vi "cg_Brent Search Powell.vi"(1 "p":dbl[](array[numeric]) format="%.2f", 2 "xit":dbl[](array[numeric]) format="%.2f", 3 "ZEPS":dbl=1e-12 format="%.2e", 6 "tol":dbl=1e-06 format="%.2e", 7 "function and data":T1, 8 "error in (no error)":errorcluster, 9 "c (start)":dbl=1.0 format="%.2f", 10 "b (start)":dbl=0.5 format="%.2f", 11 "a (start)":dbl format="%.2f") -> (0 "error out":errorcluster, 4 "u":dbl=1.5920119327128747e-12 format="%.2f", 5 "number of function calls":i32)   [LabVIEW 2010, in "NI_Gmath.lvlib"]
uses:
  NI_Gmath.lvlib
  ucno_user function ref and data.ctl
  ucno_user objective function ref.ctl
panel:
  in  "fx":dbl=3.25 format="%.2f"
  in  "fw":dbl=2.000000000005184 format="%.2f"
  in  "fv":dbl=2.000000000008388 format="%.2f"
  in  "fu":dbl=2.000000000003184 format="%.2f"
  in  "e":dbl format="%.2f"
  in  "b":dbl format="%.2f"
  in  "a":dbl format="%.2f"
  in  "x":dbl=0.5 format="%.2f"
  in  "w":dbl=2.5920145247273993e-12 format="%.2f"
  in  "v":dbl=4.1939676003423364e-12 format="%.2f"
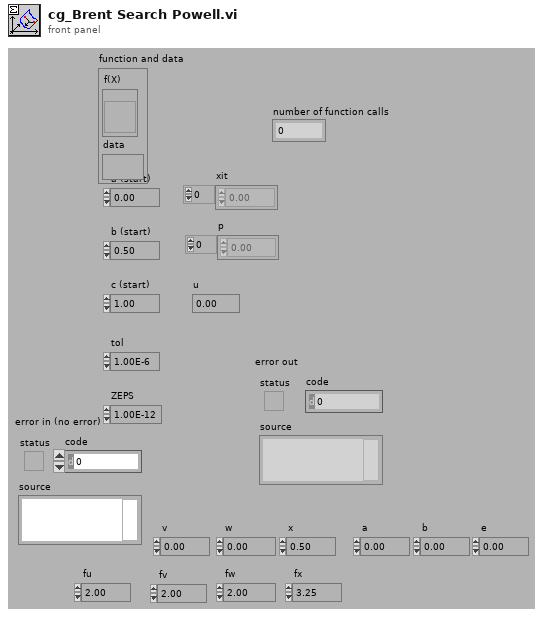
[diagram p1: front panel]
types:
  T1 = typedef "NI_Gmath.lvlib/ucno_user function ref and data.ctl" = cluster{"f(X)":T2, "data":variant}
  T2 = typedef "NI_Gmath.lvlib/ucno_user objective function ref.ctl" = refnum<vi>
  T3 = cluster{"objective function":bool, "gradient":bool}
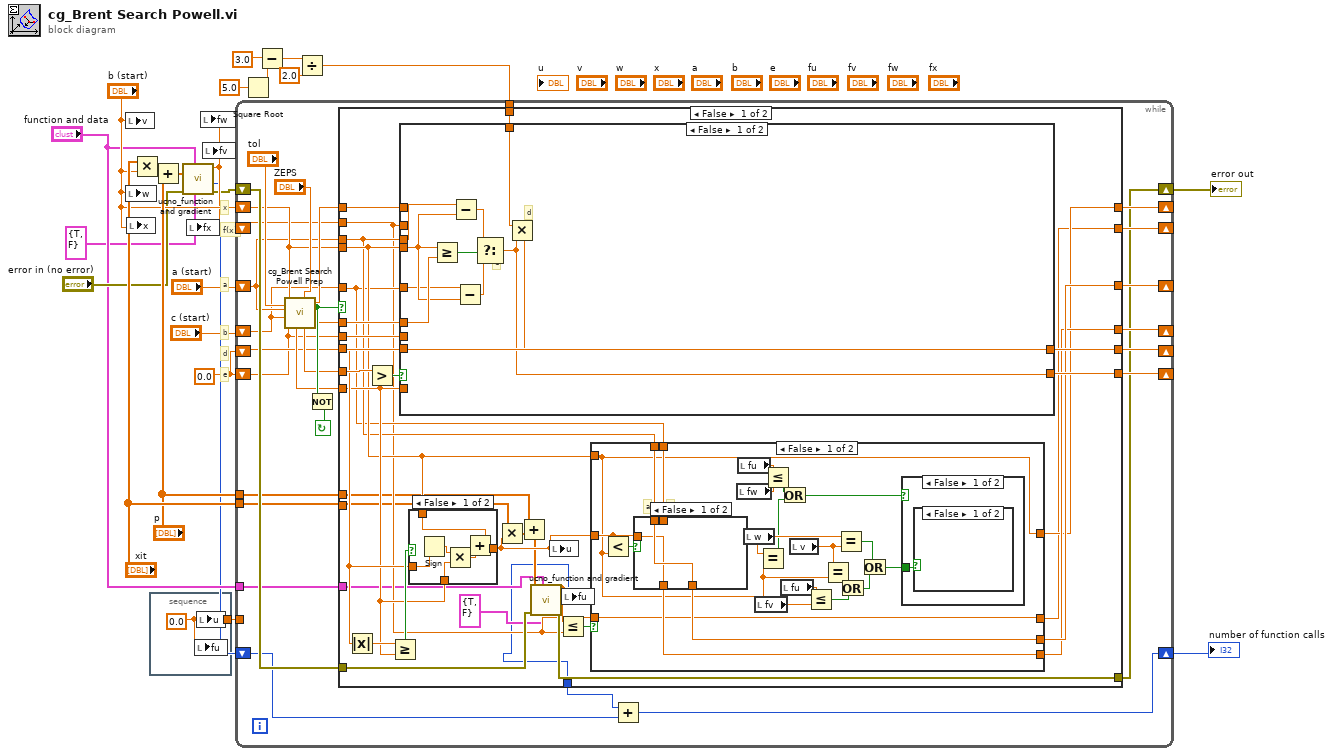
[diagram p0: block diagram]
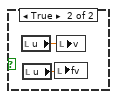
[diagram p2: hidden frame]
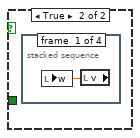
[diagram p3: hidden frame]
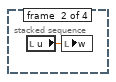
[diagram p4: hidden frame]
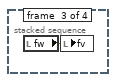
[diagram p5: hidden frame]
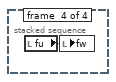
[diagram p6: hidden frame]
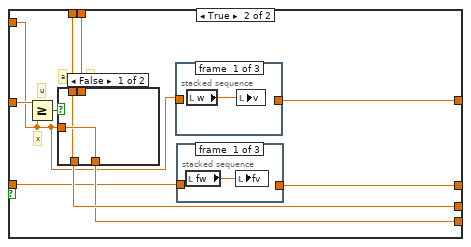
[diagram p8: hidden frame]
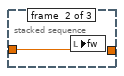
[diagram p9: hidden frame]
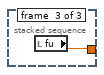
[diagram p10: hidden frame]
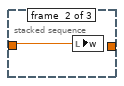
[diagram p11: hidden frame]
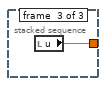
[diagram p12: hidden frame]
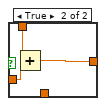
[diagram p14: hidden frame]
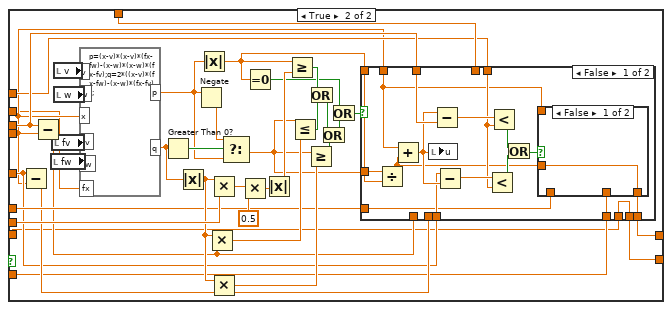
[diagram p15: hidden frame]
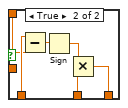
[diagram p16: hidden frame]
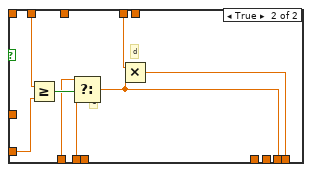
[diagram p17: hidden frame]
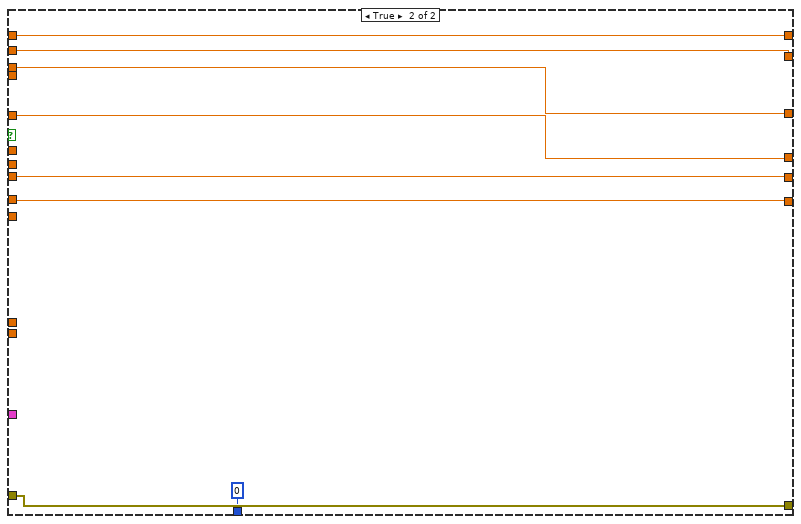
[diagram p18: hidden frame]
diagram:
  w16 = 0.0
  # "d"
  # "e"
  # "f(x)"
  # "x"
  # "b"
  # "a"
  n1 = local write "v"("b (start)") -> ()
  n2 = local write "w"("b (start)") -> ()
  n3 = local write "x"("b (start)") -> ()
  n4 = Multiply(x="xit", y="b (start)") -> (x*y=w15:dbl[])
  n5 = stacked-sequence {
    tunnel: [w24] -> w8
    frame #0 {
      w24 = 0.0
      n6 = local write "fu"(w24) -> ()
      n7 = local write "u"(w24) -> ()
    }
  }
  n8 = Add(x=w15, y="p") -> (x+y=w14:dbl[])
  n9 = call "ucno_function and gradient.vi"("output control"=T3 {"objective function"=TRUE, "gradient"=FALSE}, "function and data"="function and data", "error in (no error)"="error in (no error)", "X"=w14) -> ("error out"=w6:errorcluster, "number of function calls"=w2:i32, "f(X)"=w9:dbl)  [unwired: 4 in, 1 out]
  n10 = local write "fx"(w9) -> ()
  n11 = local write "fw"(w9) -> ()
  n12 = local write "fv"(w9) -> ()
  n13 = Square Root(x=5.0) -> (sqrt(x)=w21:dbl)
  n14 = Subtract(x=3.0, y=w21) -> (x-y=w20:dbl)
  n15 = Divide(x=w20, y=2.0) -> (x/y=w17:dbl)
  n16 = while {
    tunnel: w8 -> [_]
    tunnel: "p" -> [w31]
    tunnel: "xit" -> [w30]
    shift-left: w16 -> [w37]
    shift-right: [w38] -> _
    tunnel: w17 -> [w40]
    shift-left: w16 -> [w36]
    shift-right: [w39] -> _
    shift-left: w9 -> [w44]
    shift-right: [w32] -> _
    shift-left: "b (start)" -> [w49]
    shift-right: [w33] -> _
    shift-left: "c (start)" -> [w41]
    shift-right: [w34] -> _
    shift-left: "a (start)" -> [w42]
    shift-right: [w35] -> _
    shift-right: [w29] -> w5
    shift-left: w6 -> [w53]
    tunnel: "function and data" -> [w28]
    shift-right: [w25] -> w1
    shift-left: w2 -> [w26]
    stop <- w47 continue-if-true
    n17 = call "cg_Brent Search Powell Prep.vi"("ZEPS"="ZEPS", "e"=w36, "c (start)"=w41, "tol"="tol", "a (start)"=w42, "b (start)"=w49) -> ("value a"=w43:dbl, "value b"=w46:dbl, "convergence?"=w48:bool, "tol2"=w50:dbl, "value c"=w45:dbl)
    n18 = Not(x=w48) -> (.not. x?=w47:bool)
    n19 = case shown="False" w48 {
      tunnel: w49 -> [w69 _]
      tunnel: w46 -> [w83 w234]
      tunnel: w45 -> [w72 _]
      tunnel: w44 -> [w62 w232]
      tunnel: w43 -> [w81 _]
      tunnel: w42 -> [w68 w231]
      tunnel: w41 -> [w67 w230]
      tunnel: w40 -> [w80 _]
      tunnel: [w79 w234] -> w39
      tunnel: [w73 w235] -> w38
      tunnel: w37 -> [w78 w235]
      tunnel: w36 -> [w77 _]
      tunnel: w50 -> [w76 w233]
      tunnel: [w66 w231] -> w35
      tunnel: [w65 w230] -> w34
      tunnel: [w64 w233] -> w33
      tunnel: [w63 w232] -> w32
      tunnel: w30 -> [w60 _]
      tunnel: w31 -> [w57 _]
      tunnel: w53 -> [w85 w229]
      tunnel: [w84 w229] -> w29
      tunnel: w28 -> [w56 _]
      tunnel: [w54 0 ("number of function calls")] -> w27
      frame False {
        n20 = Greater?(x=w83, y=w72) -> (0:w82:bool)
        n21 = case shown="False" w82 {
          tunnel: w69 -> [w153 w164]
          tunnel: w62 -> [_ w163]
          tunnel: w81 -> [w157 w176]
          tunnel: w68 -> [w152 w169]
          tunnel: w67 -> [w151 w168]
          tunnel: w80 -> [w150 w173]
          tunnel: [w149 w171] -> w79
          tunnel: [w148 w172] -> w73
          tunnel: w78 -> [_ w165]
          tunnel: w77 -> [_ w189]
          tunnel: w76 -> [_ w167]
          tunnel: w72 -> [_ w166]
          frame False {
            # "d"
            # "e"
            n22 = Greater Or Equal?(x=w153, y=w157) -> (x >= y?=w156:bool)
            n23 = Subtract(x=w152, y=w153) -> (x-y=w154:dbl)
            n24 = Subtract(x=w151, y=w153) -> (x-y=w155:dbl)
            n25 = Select(t=w154, s=w156, f=w155) -> (s? t:f=w149:dbl)
            n26 = Multiply(x=w150, y=w149) -> (x*y=w148:dbl)
          }
          frame True {
            n27 = Subtract(x=w168, y=w164) -> (x-y=w174:dbl)
            n28 = Subtract(x=w169, y=w164) -> (x-y=w175:dbl)
            n29 = local read "fw"() -> (w192:dbl)
            n30 = local read "fv"() -> (w193:dbl)
            n31 = local read "v"() -> (w195:dbl)
            n32 = local read "w"() -> (w194:dbl)
            n33 = formula code="p=(x-v)*(x-v)*(fx-fw)-(x-w)*(x-w)*(fx-fv);q=2*((x-v)*(fx-fw)-(x-w)*(fx-fv));"("v"=w195, "w"=w194, "x"=w164, "fv"=w193, "fw"=w192, "fx"=w163) -> ("p"=w159:dbl, "q"=w184:dbl)
            n34 = Greater Than 0?(x=w184) -> (x > 0?=w191:bool)
            n35 = Absolute Value(x=w184) -> (abs(x)=w183:dbl)
            n36 = Negate(x=w159) -> (-x=w190:dbl)
            n37 = Absolute Value(x=w159) -> (abs(x)=w158:dbl)
            n38 = Multiply(x=w183, y=w175) -> (x*y=w182:dbl)
            n39 = Multiply(x=w183, y=w189) -> (x*y=w188:dbl)
            n40 = Multiply(x=w183, y=w174) -> (x*y=w181:dbl)
            n41 = Select(t=w190, s=w191, f=w159) -> (s? t:f=w170:dbl)
            n42 = Multiply(x=w188, y=0.5) -> (x*y=w186:dbl)
            n43 = Equal To 0?(x=w158) -> (x = 0?=w161:bool)
            n44 = Absolute Value(x=w186) -> (abs(x)=w185:dbl)
            n45 = Greater Or Equal?(x=w158, y=w185) -> (x >= y?=w180:bool)
            n46 = Less Or Equal?(x=w170, y=w182) -> (x <= y?=w179:bool)
            n47 = Greater Or Equal?(x=w170, y=w181) -> (x >= y?=w177:bool)
            n48 = Or(x=w180, y=w179) -> (x .or. y?=w178:bool)
            n49 = Or(x=w178, y=w177) -> (x .or. y?=w162:bool)
            n50 = Or(x=w161, y=w162) -> (x .or. y?=w160:bool)
            n51 = case shown="False" w160 {
              tunnel: w164 -> [w199 w226]
              tunnel: w176 -> [w200 w225]
              tunnel: w175 -> [_ w224]
              tunnel: w174 -> [_ w223]
              tunnel: w173 -> [_ w222]
              tunnel: [w197 w221] -> w172
              tunnel: [w196 w220] -> w171
              tunnel: w170 -> [w212 _]
              tunnel: w158 -> [w211 _]
              tunnel: w169 -> [w210 _]
              tunnel: w168 -> [w208 _]
              tunnel: w167 -> [w205 _]
              tunnel: w166 -> [w198 _]
              tunnel: w165 -> [w196 _]
              frame False {
                n52 = Divide(x=w212, y=w211) -> (x/y=w201:dbl)
                n53 = Add(x=w199, y=w201) -> (x+y=w209:dbl)
                n54 = local write "u"(w209) -> ()
                n55 = Subtract(x=w209, y=w210) -> (x-y=w207:dbl)
                n56 = Subtract(x=w208, y=w209) -> (x-y=w206:dbl)
                n57 = Less?(x=w206, y=w205) -> (x < y?=w203:bool)
                n58 = Less?(x=w207, y=w205) -> (x < y?=w204:bool)
                n59 = Or(x=w204, y=w203) -> (x .or. y?=w202:bool)
                n60 = case shown="False" w202 {
                  tunnel: w201 -> [w213 _]
                  tunnel: w200 -> [_ w219]
                  tunnel: w199 -> [_ w218]
                  tunnel: w198 -> [_ w215]
                  tunnel: [w213 w214] -> w197
                  frame False {
                  }
                  frame True {
                    n61 = Subtract(x=w219, y=w218) -> (x-y=w217:dbl)
                    n62 = Sign(1:w217) -> (0:w216:dbl)
                    n63 = Multiply(x=w216, y=w215) -> (x*y=w214:dbl)
                  }
                }
              }
              frame True {
                # "d"
                # "e"
                n64 = Greater Or Equal?(x=w226, y=w225) -> (x >= y?=w227:bool)
                n65 = Select(t=w224, s=w227, f=w223) -> (s? t:f=w220:dbl)
                n66 = Multiply(x=w222, y=w220) -> (x*y=w221:dbl)
              }
            }
          }
        }
        n67 = Absolute Value(x=w73) -> (abs(x)=w74:dbl)
        n68 = Greater Or Equal?(x=w74, y=w72) -> (x >= y?=w75:bool)
        n69 = case shown="False" w75 {
          tunnel: w73 -> [w144 w147]
          tunnel: w69 -> [w140 w146]
          tunnel: w72 -> [w142 _]
          tunnel: [w139 w145] -> w61
          frame False {
            n70 = Sign(1:w144) -> (0:w143:dbl)
            n71 = Multiply(x=w143, y=w142) -> (x*y=w141:dbl)
            n72 = Add(x=w140, y=w141) -> (x+y=w139:dbl)
          }
          frame True {
            n73 = Add(x=w146, y=w147) -> (x+y=w145:dbl)
          }
        }
        n74 = Multiply(x=w60, y=w61) -> (x*y=w59:dbl[])
        n75 = Add(x=w57, y=w59) -> (x+y=w58:dbl[])
        n76 = call "ucno_function and gradient.vi"("output control"=T3 {"objective function"=TRUE, "gradient"=FALSE}, "function and data"=w56, "error in (no error)"=w85, "X"=w58) -> ("error out"=w84:errorcluster, "number of function calls"=w54:i32, "f(X)"=w71:dbl)  [unwired: 4 in, 1 out]
        n77 = local write "u"(w61) -> ()
        n78 = Less Or Equal?(x=w71, y=w62) -> (x <= y?=w70:bool)
        n79 = local write "fu"(w71) -> ()
        n80 = case shown="False" w70 {
          tunnel: w61 -> [w104 w128]
          tunnel: w69 -> [w87 w122]
          tunnel: w68 -> [w106 w126]
          tunnel: w67 -> [w105 w125]
          tunnel: [w102 w124] -> w66
          tunnel: [w103 w123] -> w65
          tunnel: [w87 w121] -> w64
          tunnel: [w86 w120] -> w63
          tunnel: w62 -> [w86 w119]
          frame False {
            # "b"
            # "a"
            n81 = Less?(x=w104, y=w87) -> (x < y?=w107:bool)
            n82 = case shown="False" w107 {
              tunnel: w106 -> [w116 _]
              tunnel: w105 -> [_ w117]
              tunnel: [w116 w118] -> w102
              tunnel: w104 -> [w115 w118]
              tunnel: [w115 w117] -> w103
              frame False {
              }
              frame True {
              }
            }
            n83 = local read "fw"() -> (w100:dbl)
            n84 = local read "fu"() -> (w101:dbl)
            n85 = local read "w"() -> (w99:dbl)
            n86 = local read "fv"() -> (w95:dbl)
            n87 = Equal?(x=w99, y=w87) -> (x = y?=w98:bool)
            n88 = Less Or Equal?(x=w101, y=w100) -> (x <= y?=w97:bool)
            n89 = Or(x=w97, y=w98) -> (x .or. y?=w96:bool)
            n90 = local read "fu"() -> (w94:dbl)
            n91 = local read "v"() -> (w91:dbl)
            n92 = Less Or Equal?(x=w94, y=w95) -> (x <= y?=w92:bool)
            n93 = Equal?(x=w91, y=w87) -> (x = y?=w93:bool)
            n94 = Equal?(x=w99, y=w91) -> (x = y?=w90:bool)
            n95 = Or(x=w93, y=w92) -> (x .or. y?=w89:bool)
            n96 = Or(x=w90, y=w89) -> (x .or. y?=w88:bool)
            n97 = case shown="False" w96 {
              tunnel: w88 -> [w108 _]
              frame False {
                n98 = case shown="False" w108 {
                  frame False {
                  }
                  frame True {
                    n99 = local read "u"() -> (w110:dbl)
                    n100 = local read "u"() -> (w109:dbl)
                    n101 = local write "fv"(w109) -> ()
                    n102 = local write "v"(w110) -> ()
                  }
                }
              }
              frame True {
                n103 = stacked-sequence {
                  frame #0 {
                    n104 = local read "v"() -> (w111:dbl)
                    n105 = local write "w"(w111) -> ()
                  }
                  frame #1 {
                    n106 = local read "u"() -> (w112:dbl)
                    n107 = local write "w"(w112) -> ()
                  }
                  frame #2 {
                    n108 = local read "fw"() -> (w113:dbl)
                    n109 = local write "fv"(w113) -> ()
                  }
                  frame #3 {
                    n110 = local read "fu"() -> (w114:dbl)
                    n111 = local write "fw"(w114) -> ()
                  }
                }
              }
            }
          }
          frame True {
            # "b"
            # "a"
            # "u"
            # "x"
            n112 = Greater Or Equal?(x=w128, y=w122) -> (x >= y?=w127:bool)
            n113 = case shown="False" w127 {
              tunnel: w126 -> [w135 _]
              tunnel: w125 -> [_ w137]
              tunnel: [w135 w138] -> w124
              tunnel: w122 -> [w136 w138]
              tunnel: [w136 w137] -> w123
              frame False {
              }
              frame True {
              }
            }
            n114 = stacked-sequence {
              tunnel: w122 -> [_ w133 _]
              tunnel: [_ _ w134] -> w121
              frame #0 {
                n115 = local read "w"() -> (w132:dbl)
                n116 = local write "v"(w132) -> ()
              }
              frame #1 {
                n117 = local write "w"(w133) -> ()
              }
              frame #2 {
                n118 = local read "u"() -> (w134:dbl)
              }
            }
            n119 = stacked-sequence {
              tunnel: w119 -> [_ w130 _]
              tunnel: [_ _ w131] -> w120
              frame #0 {
                n120 = local read "fw"() -> (w129:dbl)
                n121 = local write "fv"(w129) -> ()
              }
              frame #1 {
                n122 = local write "fw"(w130) -> ()
              }
              frame #2 {
                n123 = local read "fu"() -> (w131:dbl)
              }
            }
          }
        }
      }
      frame True {
      }
    }
    n124 = Add(x=w27, y=w26) -> (x+y=w25:i32)
  }
  "error out" <- w5
  "number of function calls" <- w1
